vi "Test Config Iface Default Boolean.vi"(8 "error in (no error)":errorcluster, 11 "Test Case In":refnum<class "Configuration Interface Test.lvclass">) -> (0 "error out":errorcluster, 3 "Test Case Out":refnum<class "Configuration Interface Test.lvclass">)   [LabVIEW 2020, in "Configuration Interface Test.lvclass"]
uses:
  Configuration Interface Test.lvclass
  C:/Program Files (x86)/National Instruments/LabVIEW 2020/vi.lib/Astemes/LUnit/Test Case.lvclass
  source/Framework/Configuration/Configuration.lvclass
  <vilib>/Astemes/LUnit/Test Case.lvclass/Test Case.ctl
  <vilib>/Astemes/LUnit/LUnit Assertion Result.lvclass/LUnit Assertion Result.ctl
  <vilib>/Astemes/LUnit/LUnit Test Case Result.lvclass/LUnit Test Case Result.ctl
  <vilib>/Astemes/LUnit/LUnit Method Result.lvclass/LUnit Method Result.ctl
  74dde7e8-af02-4f55-b1fe-f43fb403aab3.vi
  <vilib>/Astemes/LUnit/Palette/Pass.vi
  <vilib>/Astemes/LUnit/Palette/Fail.vi
  <vilib>/Astemes/LUnit/Compare Variants.vi
  <vilib>/Astemes/LUnit/Describe Comparison.vi
  <vilib>/Astemes/LUnit/Set Assertion Type.vi
  <vilib>/Astemes/LUnit/Add test result.vi
  <vilib>/Astemes/LUnit/LUnit Write Message.vi
  <vilib>/Astemes/LUnit/LUnit Write Description.vi
  <vilib>/Astemes/LUnit/LUnit Write Skipped.vi
  <vilib>/Astemes/LUnit/LUnit Write Passed.vi
  <vilib>/Astemes/LUnit/Variant to string.vi
  <vilib>/Astemes/LUnit/LUnit Write Assertion Type.vi
  <vilib>/Astemes/LUnit/LUnit Record Assertion Result.vi
  <vilib>/Astemes/LUnit/LUnit Aggregate Assertion Results.vi
  <vilib>/Astemes/LUnit/Assertion Result/LUnit Read Status.vi
  <vilib>/Astemes/LUnit/LUnit Read Message.vi
  <vilib>/Astemes/LUnit/LUnit Read Description.vi
  <vilib>/Astemes/LUnit/Method Result/LUnit Merge Status.vi
  <vilib>/Astemes/LUnit/LUnit Concatenate result strings.vi
  <vilib>/Utility/Data Type/Get Type Information.vi
  <vilib>/Utility/LVClass/Get LV Class Name.vi
  <vilib>/Astemes/LUnit/LUnit Assertion Result.lvclass
  <vilib>/Astemes/LUnit/Test Case.lvclass
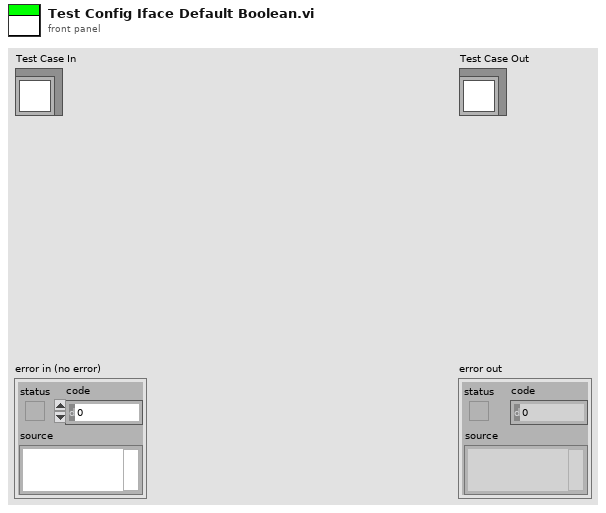
[diagram p1: front panel]
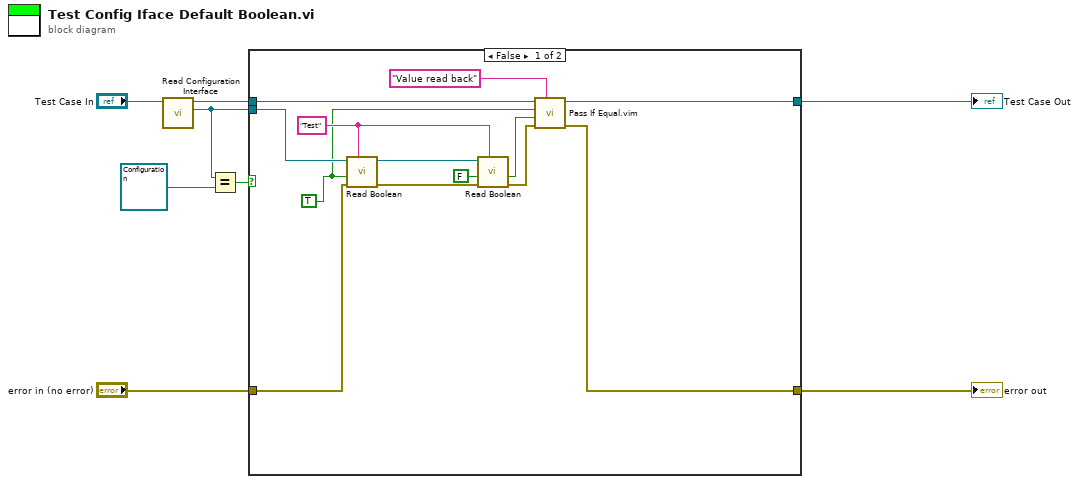
[diagram p0: block diagram]
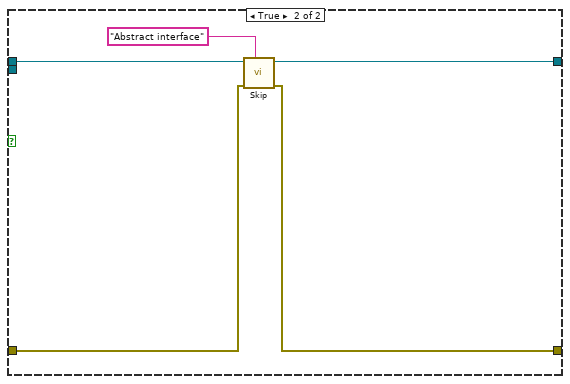
[diagram p2: hidden frame]
diagram:
  n1 = call "Read Configuration Interface.vi"("Configuration Interface Test In"="Test Case In") -> ("Configuration"=w3:refnum<class "Configuration.lvclass">, "Configuration Interface Test Out"=w6:refnum<class "Configuration Interface Test.lvclass">)  [unwired: 9 in]
  n2 = Equal?(x=w3, y=refnum<class "Configuration.lvclass"> refnum ("Configuration")) -> (x = y?=w1:bool)
  n3 = case shown="False" w1 {
    tunnel: [w17 w23] -> w7
    tunnel: w6 -> [w16 w26]
    tunnel: [w15 w25] -> w5
    tunnel: "error in (no error)" -> [w13 w24]
    tunnel: w3 -> [w12 _]
    frame False {
      w10 = TRUE ("Value")
      w19 = "Test" ("key")
      n4 = call-dynamic "Read Boolean.vi"("key"=w19, "error in (no error)"=w13, "default value"=w10, "Configuration In"=w12) -> ("error out"=w20:errorcluster, "Configuration Out"=w21:refnum<class "Configuration.lvclass">)  [unwired: 5 in, 1 out]
      n5 = call-dynamic "Read Boolean.vi"("key"=w19, "error in (no error)"=w20, "default value"=FALSE, "Configuration In"=w21) -> ("error out"=w14:errorcluster, "value"=w9:bool)  [unwired: 5 in, 1 out]
      n6 = call "Pass If Equal.vim"("Description"="Value read back", "error in (no error)"=w14, "Actual"=w9, "Expected"=w10, "LUnit Test Case In"=w16) -> ("error out"=w17:errorcluster, "LUnit Test Case Out"=w15:refnum<class "Configuration Interface Test.lvclass">)  [unwired: 5 in]
    }
    frame True {
      n7 = call <vilib>:"Skip.vi"("Description"="Abstract interface", "error in (no error)"=w24, "LUnit Test Case In"=w26) -> ("error out"=w23:errorcluster, "LUnit Test Case Out"=w25:refnum<class "Configuration Interface Test.lvclass">)  [unwired: 7 in]
    }
  }
  "error out" <- w7
  "Test Case Out" <- w5
